vi "replaceTabElement.vi"(8 "error in (no error)":errorcluster, 9 "replaceWith":string, 10 "replaceElementLabeled":string, 11 "Tab ref in":refnum<vi>) -> (0 "error out":errorcluster, 3 "Tab ref out":refnum<vi>)   [LabVIEW 2011, in "Views.lvlib" / "Camera.lvlib" / "andorSettingsViewer.lvclass"]
uses:
  CameraSettingsViewer/andorSettingsViewer.lvclass
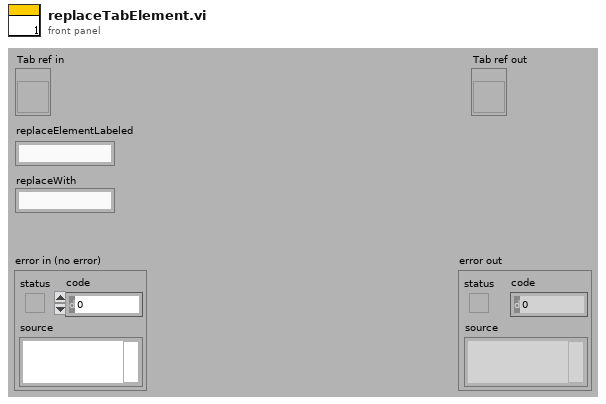
[diagram p1: front panel]
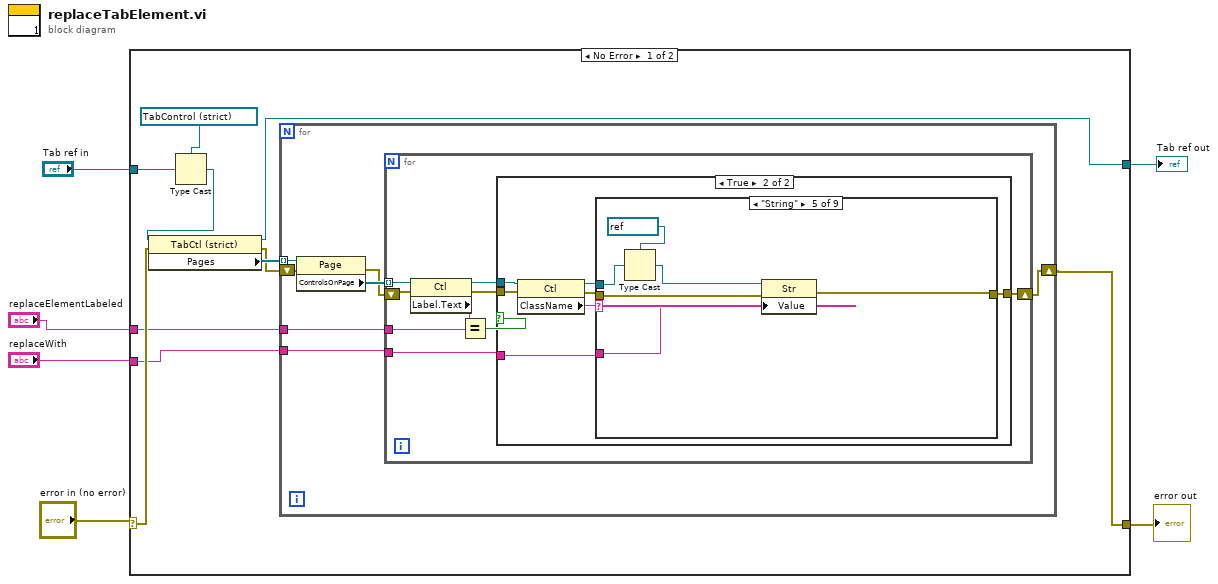
[diagram p0: block diagram]
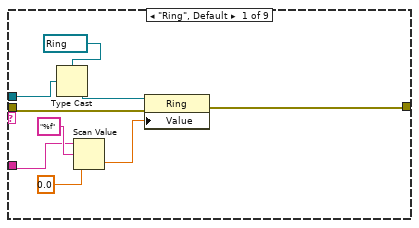
[diagram p3: hidden frame]
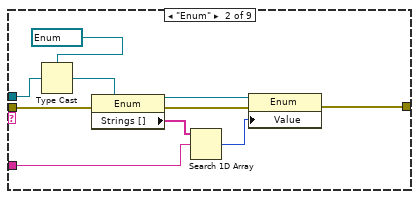
[diagram p4: hidden frame]
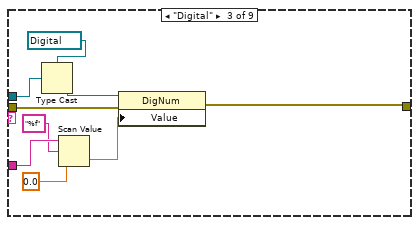
[diagram p5: hidden frame]
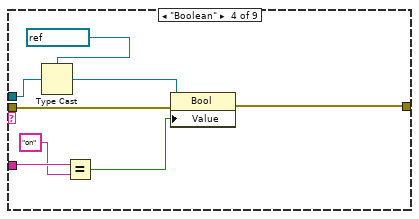
[diagram p6: hidden frame]
diagram:
  n1 = case shown="No Error" "error in (no error)" {
    selector: "error in (no error)" -> [w14 w88]
    tunnel: [w9 w88] -> w5
    tunnel: "replaceElementLabeled" -> [w13 _]
    tunnel: "replaceWith" -> [w12 _]
    tunnel: "Tab ref in" -> [w11 w87]
    tunnel: [w7 w87] -> w1
    frame No Error {
      n2 = Type Cast(type=refnum<vi> refnum ("Tab Control"), x=w11) -> (*(type *) &x=w8:refnum<vi>)
      n3 = property class="TabCtl (strict)"(reference=w8, error in=w14) -> (reference out=w7:refnum<vi>, error out=w15:errorcluster, "Pages"=w16:refnum<vi>[])
      n4 = for {
        tunnel: w16 -> [w23] mode=indexing
        tunnel: w13 -> [w21]
        tunnel: w12 -> [w20]
        shift-right: [w18] -> w9
        shift-left: w15 -> [w19]
        n5 = property class="Page"(reference=w23, error in=w19) -> (error out=w17:errorcluster, "ControlsOnPage"=w22:refnum<vi>[])  [unwired: 1 out]
        n6 = for {
          tunnel: w22 -> [w31] mode=indexing
          tunnel: w21 -> [w29]
          tunnel: w20 -> [w28]
          shift-right: [w25] -> w18
          shift-left: w17 -> [w26]
          n7 = property class="Ctl"(reference=w31, error in=w26) -> (reference out=w24:refnum<vi>, error out=w27:errorcluster, "Label.Text"=w32:string)
          n8 = Equal?(x=w32, y=w29) -> (x = y?=w30:bool)
          n9 = case shown="True" w30 {
            tunnel: w28 -> [_ w39]
            tunnel: [w33 w35] -> w25
            tunnel: w27 -> [w33 w36]
            tunnel: w24 -> [_ w34]
            frame False {
            }
            frame True {
              n10 = property class="Ctl"(reference=w34, error in=w36) -> (reference out=w40:refnum<vi>, error out=w37:errorcluster, "ClassName"=w38:string)
              n11 = case shown="\"String\"" w38 {
                tunnel: w40 -> [w44 w56 w68 w76 w82 _ _ _ _]
                tunnel: w39 -> [w42 w55 w64 w74 w81 _ _ _ _]
                tunnel: w37 -> [w43 w54 w66 w71 w80 w83 w84 w85 w86]
                tunnel: [w41 w52 w60 w69 w77 w83 w84 w85 w86] -> w35
                frame "Ring", Default {
                  n12 = Type Cast(type=refnum<vi> refnum ("id"), x=w44) -> (*(type *) &x=w49:refnum<vi>)
                  n13 = Scan Value(string=w42, format string="%f", default (0 dbl)=0.0) -> (value=w46:dbl)  [unwired: 1 out]
                  n14 = property class="Ring"(reference=w49, error in=w43, "Value"=w46) -> (error out=w41:errorcluster)  [unwired: 1 out]
                }
                frame "Enum" {
                  n15 = Type Cast(type=refnum<vi> refnum ("id"), x=w56) -> (*(type *) &x=w57:refnum<vi>)
                  n16 = property class="Enum"(reference=w57, error in=w54) -> (reference out=w58:refnum<vi>, error out=w59:errorcluster, "Strings []"=w51:string[])
                  n17 = Search 1D Array(1D array=w51, element=w55) -> (index of element=w50:i32)  [unwired: 1 in]
                  n18 = property class="Enum"(reference=w58, error in=w59, "Value"=w50) -> (error out=w52:errorcluster)  [unwired: 1 out]
                }
                frame "Digital" {
                  n19 = Type Cast(type=refnum<vi> refnum ("id"), x=w68) -> (*(type *) &x=w67:refnum<vi>)
                  n20 = Scan Value(string=w64, format string="%f", default (0 dbl)=0.0) -> (value=w62:dbl)  [unwired: 1 out]
                  n21 = property class="DigNum"(reference=w67, error in=w66, "Value"=w62) -> (error out=w60:errorcluster)  [unwired: 1 out]
                }
                frame "Boolean" {
                  n22 = Type Cast(type=refnum<vi> refnum ("Boolean"), x=w76) -> (*(type *) &x=w75:refnum<vi>)
                  n23 = Equal?(x=w74, y="on") -> (x = y?=w72:bool)
                  n24 = property class="Bool"(reference=w75, error in=w71, "Value"=w72) -> (error out=w69:errorcluster)  [unwired: 1 out]
                }
                frame "String" {
                  n25 = Type Cast(type=refnum<vi> refnum ("String"), x=w82) -> (*(type *) &x=w78:refnum<vi>)
                  n26 = property class="Str"(reference=w78, error in=w80, "Value"=w81) -> (error out=w77:errorcluster)  [unwired: 1 out]
                }
                frame "Path" {
                }
                frame "Cluster" {
                }
                frame "Array" {
                }
                frame "MulticolumnListbox" {
                }
              }
            }
          }
        }
      }
    }
    frame Error {
    }
  }
  "error out" <- w5
  "Tab ref out" <- w1
